vi "Image Loader.vi"() -> ()   [LabVIEW 2015]
uses:
  <vilib>/picture/picture.llb/imagedata.ctl
panel:
  out "image data":T1
  out "Image":picture
  in  "Image Path":path
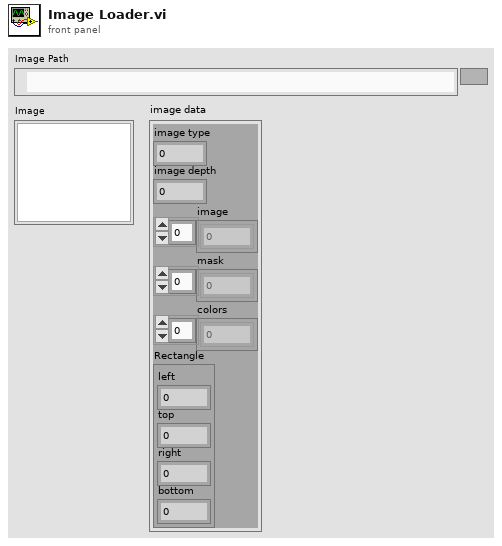
[diagram p1: front panel]
types:
  T1 = typedef "imagedata.ctl" = cluster{"image type":i32, "image depth":i32, "image":u8[], "mask":u8[], "colors":u32[], "Rectangle":cluster{"left":i16, "top":i16, "right":i16, "bottom":i16}}
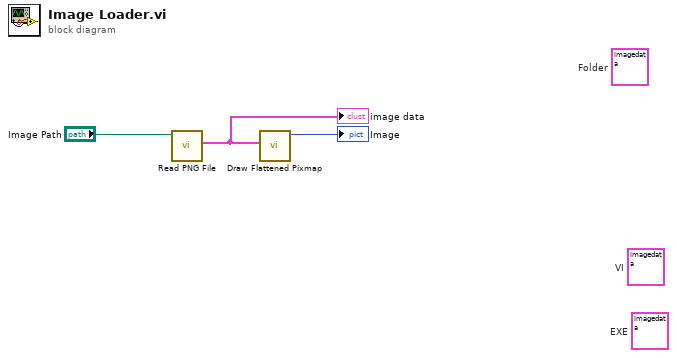
[diagram p0: block diagram]
diagram:
  (unwired) T1 {"image type"=0, "image depth"=24, "image"=[132, 132, 132, 132, 132, 132, 132, 132, 132, 132, 132, 132, 132, 132, 132, 132, 132, 132, 132, 132, 132, 132, 132, 132, 132, 132, 132, 132, 132, 132, 132, 132, 132, 132, 132, 132, 132, 132, 132, 132, 132, 132, 132, 132, 132, 132, 132, 132, 132, 132, 132, 198, 198, 198, 198, 198, 198, 198, 198, 198, 198, 198, 198, 198, 198, 198, 198, 198, 198, 198, 198, 198, 198, 198, 198, 198, 198, 198, 198, 198, 198, 198, 198, 198, 198, 198, 198, 198, 198, 198, 132, 132, 132, 0, 0, 0, 132, 132, 132, 198, 198, 198, 0, 0, 189, 0, 0, 189, 0, 0, 189, 0, 0, 189, 0, 0, 189, 0, 0, 189, 0, 0, 189, 0, 0, 189, 0, 0, 189, 0, 0, 189, 0, 0, 189, 0, 0, 189, 132, 132, 132, 0, 0, 0, 132, 132, 132, 198, 198, 198, 0, 0, 189, 0, 0, 189, 0, 0, 189, 0, 0, 189, 0, 0, 189, 0, 0, 189, 255, 255, 255, 0, 0, 0, 255, 255, 255, 0, 0, 0, 255, 255, 255, 0, 0, 0, 132, 132, 132, 0, 0, 0, 132, 132, 132, 198, 198, 198, 132, 132, 132, 132, 132, 132, 132, 132, 132, 132, 132, 132, 132, 132, 132, 132, 132, 132, 132, 132, 132, 132, 132, 132, 132, 132, 132, 132, 132, 132, 132, 132, 132, 132, 132, 132, 132, 132, 132, 0, 0, 0, 132, 132, 132, 198, 198, 198, 255, 255, 255, 255, 255, 255, 255, 255, 255, 255, 255, 255, 255, 255, 255, 255, 255, 255, 255, 255, 255, 255, 255, 255, 255, 255, 255, 255, 255, 255, 255, 255, 255, 255, 255, 255, 132, 132, 132, 0, 0, 0, 132, 132, 132, 198, 198, 198, 255, 255, 255, 255, 255, 255, 255, 255, 255, 255, 255, 255, 255, 255, 255, 255, 255, 255, 255, 255, 255, 255, 255, 255, 255, 255, 255, 255, 255, 255, 255, 255, 255, 255, 255, 255, 132, 132, 132, 0, 0, 0, 132, 132, 132, 198, 198, 198, 255, 255, 255, 255, 255, 255, 255, 255, 255, 255, 255, 255, 255, 255, 255, 255, 255, 255, 255, 255, 255, 255, 255, 255, 255, 255, 255, 255, 255, 255, 255, 255, 255, 255, 255, 255, 132, 132, 132, 0, 0, 0, 132, 132, 132, 198, 198, 198, 255, 255, 255, 255, 255, 255, 255, 255, 255, 255, 255, 255, 255, 255, 255, 255, 255, 255, 255, 255, 255, 255, 255, 255, 255, 255, 255, 255, 255, 255, 255, 255, 255, 255, 255, 255, 132, 132, 132, 0, 0, 0, 132, 132, 132, 198, 198, 198, 255, 255, 255, 255, 255, 255, 255, 255, 255, 255, 255, 255, 255, 255, 255, 255, 255, 255, 255, 255, 255, 255, 255, 255, 255, 255, 255, 255, 255, 255, 255, 255, 255, 255, 255, 255, 132, 132, 132, 0, 0, 0, 132, 132, 132, 198, 198, 198, 255, 255, 255, 255, 255, 255, 255, 255, 255, 255, 255, 255, 255, 255, 255, 255, 255, 255, 255, 255, 255, 255, 255, 255, 255, 255, 255, 255, 255, 255, 255, 255, 255, 255, 255, 255, 132, 132, 132, 0, 0, 0, 132, 132, 132, 198, 198, 198, 255, 255, 255, 255, 255, 255, 255, 255, 255, 255, 255, 255, 255, 255, 255, 255, 255, 255, 255, 255, 255, 255, 255, 255, 255, 255, 255, 255, 255, 255, 255, 255, 255, 255, 255, 255, 132, 132, 132, 0, 0, 0, 132, 132, 132, 132, 132, 132, 132, 132, 132, 132, 132, 132, 132, 132, 132, 132, 132, 132, 132, 132, 132, 132, 132, 132, 132, 132, 132, 132, 132, 132, 132, 132, 132, 132, 132, 132, 132, 132, 132, 132, 132, 132, 132, 132, 132, 0, 0, 0, 0, 0, 0, 0, 0, 0, 0, 0, 0, 0, 0, 0, 0, 0, 0, 0, 0, 0, 0, 0, 0, 0, 0, 0, 0, 0, 0, 0, 0, 0, 0, 0, 0, 0, 0, 0, 0, 0, 0, 0, 0, 0, 0, 0, 0, 0, 0, 0], "mask"=[], "colors"=[], "Rectangle"={"left"=0, "top"=0, "right"=16, "bottom"=14}}  # EXE
  (unwired) T1 {"image type"=0, "image depth"=32, "image"=[255, 132, 170, 222, 255, 132, 170, 222, 255, 132, 170, 222, 255, 132, 170, 222, 255, 132, 170, 222, 255, 132, 170, 222, 255, 132, 170, 222, 255, 132, 170, 222, 255, 132, 170, 222, 255, 132, 170, 222, 255, 115, 130, 181, 0, 0, 0, 0, 0, 0, 0, 0, 0, 0, 0, 0, 0, 0, 0, 0, 255, 132, 154, 206, 255, 255, 255, 255, 255, 255, 255, 255, 255, 255, 255, 255, 255, 255, 255, 255, 255, 255, 255, 255, 255, 255, 255, 255, 255, 255, 255, 255, 255, 255, 255, 255, 255, 231, 243, 255, 255, 115, 130, 181, 255, 132, 170, 222, 0, 0, 0, 0, 0, 0, 0, 0, 0, 0, 0, 0, 255, 132, 154, 206, 255, 247, 251, 255, 255, 255, 255, 255, 255, 255, 251, 255, 255, 247, 247, 247, 255, 247, 247, 247, 255, 247, 247, 247, 255, 247, 247, 247, 255, 231, 243, 255, 255, 231, 243, 255, 255, 115, 130, 181, 255, 115, 130, 181, 255, 115, 130, 181, 0, 0, 0, 0, 0, 0, 0, 0, 255, 132, 154, 206, 255, 247, 251, 255, 255, 247, 251, 255, 255, 247, 243, 247, 255, 247, 243, 247, 255, 247, 243, 247, 255, 231, 243, 255, 255, 231, 243, 255, 255, 231, 243, 255, 255, 231, 243, 255, 255, 231, 243, 255, 255, 206, 211, 255, 255, 115, 121, 173, 0, 0, 0, 0, 0, 0, 0, 0, 255, 132, 158, 206, 255, 198, 199, 222, 255, 189, 186, 214, 255, 189, 186, 214, 255, 189, 186, 214, 255, 189, 186, 214, 255, 189, 186, 214, 255, 189, 186, 214, 255, 189, 186, 214, 255, 189, 186, 214, 255, 107, 109, 140, 255, 206, 211, 255, 255, 115, 121, 173, 0, 0, 0, 0, 0, 0, 0, 0, 255, 132, 154, 206, 255, 189, 186, 214, 255, 189, 178, 165, 255, 189, 178, 165, 255, 189, 178, 165, 255, 189, 178, 165, 255, 189, 178, 165, 255, 189, 178, 165, 255, 165, 162, 165, 255, 156, 154, 156, 255, 132, 134, 173, 255, 206, 211, 255, 255, 115, 121, 173, 0, 0, 0, 0, 0, 0, 0, 0, 255, 132, 150, 198, 255, 189, 186, 214, 255, 24, 142, 8, 255, 0, 16, 0, 255, 24, 121, 16, 255, 0, 0, 0, 255, 24, 125, 16, 255, 66, 73, 57, 255, 189, 178, 165, 255, 181, 170, 156, 255, 148, 142, 173, 255, 206, 211, 255, 255, 115, 121, 173, 0, 0, 0, 0, 0, 0, 0, 0, 255, 132, 150, 198, 255, 189, 186, 214, 255, 24, 134, 8, 255, 0, 16, 0, 255, 24, 121, 16, 255, 0, 12, 0, 255, 24, 121, 16, 255, 66, 89, 57, 255, 214, 178, 24, 255, 206, 199, 181, 255, 140, 138, 173, 255, 206, 211, 255, 255, 115, 121, 173, 0, 0, 0, 0, 0, 0, 0, 0, 255, 123, 138, 181, 255, 189, 186, 214, 255, 0, 16, 0, 255, 24, 121, 16, 255, 0, 16, 0, 255, 24, 121, 16, 255, 0, 12, 0, 255, 49, 73, 99, 255, 214, 178, 24, 255, 140, 130, 33, 255, 140, 130, 33, 255, 206, 211, 255, 255, 115, 121, 173, 0, 0, 0, 0, 0, 0, 0, 0, 255, 123, 134, 181, 255, 189, 186, 214, 255, 0, 0, 0, 255, 0, 121, 24, 255, 0, 0, 0, 255, 0, 121, 24, 255, 0, 4, 0, 255, 181, 174, 165, 255, 214, 182, 24, 255, 255, 255, 0, 255, 255, 255, 0, 255, 140, 130, 33, 255, 140, 130, 33, 0, 0, 0, 0, 0, 0, 0, 0, 255, 123, 130, 173, 255, 189, 186, 214, 255, 181, 178, 165, 255, 181, 178, 165, 255, 181, 178, 165, 255, 181, 178, 165, 255, 255, 0, 0, 255, 255, 0, 0, 255, 214, 182, 24, 255, 255, 255, 0, 255, 107, 101, 33, 255, 255, 255, 0, 255, 255, 255, 0, 255, 140, 130, 33, 0, 0, 0, 0, 255, 123, 125, 173, 255, 189, 186, 214, 255, 181, 178, 165, 255, 181, 178, 165, 255, 181, 178, 165, 255, 181, 178, 165, 255, 181, 178, 165, 255, 181, 178, 165, 255, 214, 182, 24, 255, 107, 101, 33, 255, 0, 0, 0, 255, 107, 101, 33, 255, 255, 255, 0, 255, 255, 0, 0, 255, 255, 0, 0, 255, 115, 121, 165, 255, 181, 182, 214, 255, 123, 121, 140, 255, 123, 121, 140, 255, 123, 121, 140, 255, 123, 121, 140, 255, 0, 0, 255, 255, 0, 0, 255, 255, 214, 182, 24, 255, 255, 255, 0, 255, 107, 101, 33, 255, 255, 255, 0, 255, 255, 255, 0, 255, 99, 93, 49, 0, 0, 0, 0, 255, 115, 121, 165, 255, 206, 211, 255, 255, 206, 211, 255, 255, 206, 211, 255, 255, 206, 211, 255, 255, 206, 211, 255, 255, 206, 211, 255, 255, 206, 211, 255, 255, 214, 182, 24, 255, 255, 255, 0, 255, 255, 255, 0, 255, 140, 130, 33, 255, 140, 130, 33, 0, 0, 0, 0, 0, 0, 0, 0, 255, 115, 121, 173, 255, 115, 121, 173, 255, 115, 121, 173, 255, 115, 121, 173, 255, 115, 121, 173, 255, 115, 121, 173, 255, 115, 121, 173, 255, 115, 121, 173, 255, 206, 182, 66, 255, 148, 134, 33, 255, 140, 130, 33, 255, 115, 121, 173, 255, 115, 121, 173, 0, 0, 0, 0, 0, 0, 0, 0], "mask"=[255, 224, 255, 240, 255, 248, 255, 248, 255, 248, 255, 248, 255, 248, 255, 248, 255, 248, 255, 248, 255, 252, 255, 254, 255, 252, 255, 248, 255, 248], "colors"=[], "Rectangle"={"left"=0, "top"=0, "right"=15, "bottom"=15}}  # VI
  (unwired) T1 {"image type"=0, "image depth"=32, "image"=array[1024 elements], "mask"=[0, 0, 60, 0, 126, 0, 255, 248, 255, 252, 255, 254, 255, 255, 255, 255, 255, 255, 255, 255, 255, 254, 255, 254, 255, 254, 127, 252, 0, 0, 0, 0], "colors"=[], "Rectangle"={"left"=0, "top"=0, "right"=16, "bottom"=16}}  # Folder
  n1 = call <vilib>:"Read PNG File.vi"("path to PNG file"="Image Path") -> ("image data"=w2:T1)  [unwired: 8 in, 2 out]
  "image data" <- w2
  n2 = call <vilib>:"Draw Flattened Pixmap.vi"("image data"=w2) -> ("new picture"=→"Image":picture)  [unwired: 8 in]
